vi "Check File Status.vi"(8 "error in":errorcluster, 11 "File in":refnum<class "File.lvclass">) -> (0 "error out":errorcluster, 3 "File out":refnum<class "File.lvclass">)   [LabVIEW 2013, in "File.lvclass"]
uses:
  File.lvclass
  File.lvclass/File.ctl
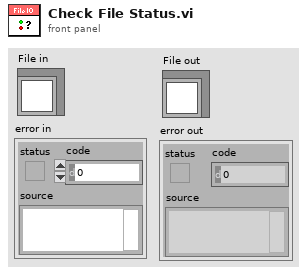
[diagram p1: front panel]
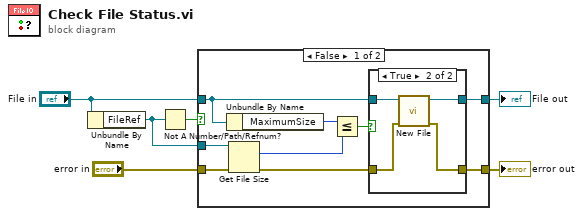
[diagram p0: block diagram]
diagram:
  n1 = Unbundle By Name("File in") -> ("FileRef"=w4:refnum<file>)
  n2 = Not A Number/Path/Refnum?(number/path/refnum=w4) -> (NaN/Path/Refnum?=w6:bool)
  n3 = case shown="False" w6 {
    tunnel: "File in" -> [w7 w23]
    tunnel: w4 -> [w15 _]
    tunnel: [w11 w23] -> w3
    tunnel: "error in" -> [w10 w22]
    tunnel: [w8 w22] -> w1
    frame False {
      n4 = Unbundle By Name(w7) -> ("MaximumSize"=w14:i64)
      n5 = Get File Size(file=w15, error in=w10) -> (size (in bytes)=w13:i64, 0:w9:errorcluster)  [unwired: 1 out]
      n6 = Less Or Equal?(x=w14, y=w13) -> (x <= y?=w12:bool)
      n7 = case shown="True" w12 {
        tunnel: w7 -> [w17 w21]
        tunnel: [w17 w20] -> w11
        tunnel: w9 -> [w16 w19]
        tunnel: [w16 w18] -> w8
        frame False {
        }
        frame True {
          n8 = call-dynamic "New File.vi"("error in"=w19, "File in"=w21) -> ("error out"=w18:errorcluster, "File out"=w20:refnum<class "File.lvclass">)  [unwired: 8 in]
        }
      }
    }
    frame True {
    }
  }
  "error out" <- w1
  "File out" <- w3
